vi "Constants.vi"() -> ()   [LabVIEW 2020, in "Ballard ARINC 429 Scripting.lvlib"]
doc: "Use this Global VI to access the GUIDs assigned to the page resources of the Custom Device."
uses:
  Ballard ARINC 429 Scripting.lvlib
panel:
  in  "Tab Control":enum32{"GUIDs", "Constants", "Properties"}(tab)=enum."Constants"
  in  "GUID.Status":string="d3f909f4-31dd-4b46-b0c0-188c355fd2ae"
  in  "GUID.Static Chan":string="0ceacc7e-2a0c-4161-94e4-a05224c7d47b"
  in  "GUID.Timestamp Channel":string="3b6787ca-0ab3-48b7-849a-2ad8b01a43ed"
  in  "GUID.Word":string="f906cc29-2aac-40b2-844c-3debd55d7c10"
  in  "GUID.Channel":string="7862A4D1-00AD-42C2-8A9F-4C525861A8AC"
  in  "GUID.Import Frames":string="0697C98A-9CCE-47AB-B6F9-386AC77E8880"
  in  "GUID.Outgoing":string="7D7F8E01-8E02-4E6A-8E22-BF1B7D107645"
  in  "GUID.Incoming":string="3098426F-4C09-481E-8916-57E537FEC0AE"
  in  "GUID.Database":string="93911212-5CC3-4FE5-877D-B534BF9C5E40"
  in  "GUID.Add Database":string="D7790871-F68E-4527-B8AD-D6388CFBE356"
  in  "GUID.Port":string="4344CD5A-2266-4D64-A775-8F5615E9A1AD"
  in  "GUID.Add Port":string="4DC2F88C-216B-4D3D-990A-E6D477C716D8"
  in  "GUID.Databases":string="5F9EF1FD-304F-4EA9-BDF8-DC215A306754"
  in  "GUID.Ports":string="879B7DAF-C156-4E60-80C7-980946E79B26"
  in  "GUID.Protocol":string="D8399BD9-D898-4CE7-A38F-CD0EDB89D6D6"
  in  "GUID.Vendor":string="2F6A7EFE-5C12-4510-A940-FB1E70DEF407"
  in  "GUID.Frame":string="8CE6E51F-BC83-4569-865F-9C808FB30A26"
  in  "GUID.Communication Bus Template":string="123EAA23-BADA-4DDC-980E-A4FC910D5182"
  in  "PXI Slot Number":string="PXI Slot Number"
  in  "Card Number":string="Card Number"
  in  "Channel":string="Channel"
  in  "Import Frames":string="Import Frames"
  in  "Frame":string="Frame"
  in  "Outgoing":string="Outgoing"
  in  "Incoming":string="Incoming"
  in  "Add Database":string="Add Database"
  in  "Database":string="Database"
  in  "Port":string="Port"
  in  "Add Port":string="Add Port"
  in  "Databases":string="Databases"
  in  "Ports":string="Ports"
  in  "Prop.PXI.Slot.Number":string="PXI Slot Number"
  in  "Prop.Initialization.Method":string="Initialization Method"
  in  "Prop.Core.Number":string="core number"
  in  "Prop.Card.Number":string="card number"
  in  "Prop.Port":string="Port"
  in  "Prop.Asynchronous.Loop.Time":string="Asynchronous Loop Time"
  in  "Prop.Word.Initial.Raw.Value":string="WordInitialRawValue"
  in  "Prop.xml.Name":string="xmlName"
  in  "Prop.Label":string="Label"
  in  "Prop.Raw.Data.Bits":string="RawData Bits"
  in  "Prop.SDI.Enabled":string="SDI_Enabled"
  in  "Prop.SDI.Value":string="SDIValue"
  in  "Prop.TxRate":string="txRate"
  in  "Prop.Transfer.Type":string="TransferType"
  in  "Prop.Default.word":string="Default word"
  in  "Prop.Encoding.Type":string="Encoding Type"
  in  "Prop.Start.Bit":string="Start Bit"
  in  "Prop.Num.Bits":string="Num Bits"
  in  "Prop.Signed?":string="Signed?"
  in  "Prop.Scale.Fac":string="ScaleFac"
  in  "Prop.Scale.Offset":string="ScaleOffset"
  in  "Prop.Unit":string="Unit"
  in  "Prop.Baud.Rate":string="Baud.Rate"
  in  "Prop.Database.Path":string="Database.Path"
  in  "Prop.Database.Name":string="Database.Name"
  in  "Prop.Frame.ID":string="Frame.ID"
  in  "Prop.Compiled.Settings":string="Compiled.Settings"
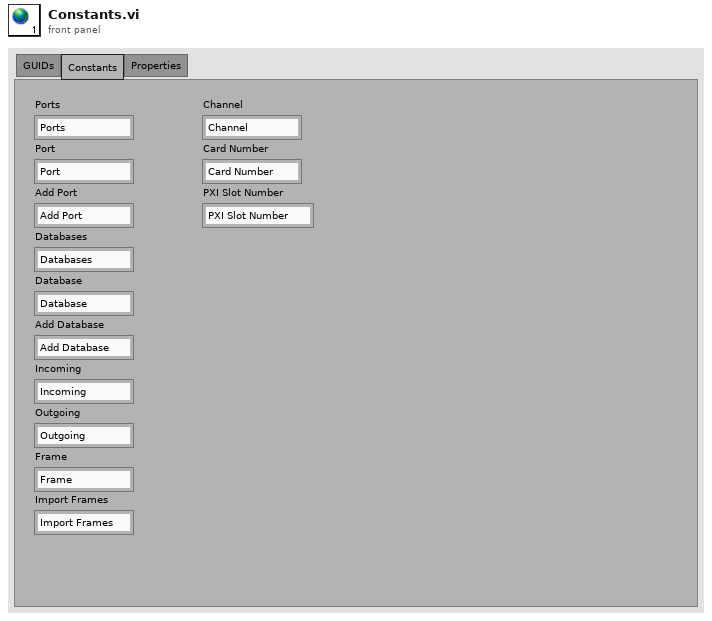
[diagram p1: front panel]
diagram:
